vi "Write Sender.vi"(8 "error in (no error)":errorcluster, 10 "Sender":string, 11 "iMessage in":refnum<class "iMessage.lvclass">) -> (0 "error out":errorcluster, 3 "iMessage out":refnum<class "iMessage.lvclass">)   [LabVIEW 2017, in "Message Interface.lvlib" / "iMessage.lvclass"]
uses:
  iMessage.lvclass
  iMessage.lvclass/iMessage.ctl
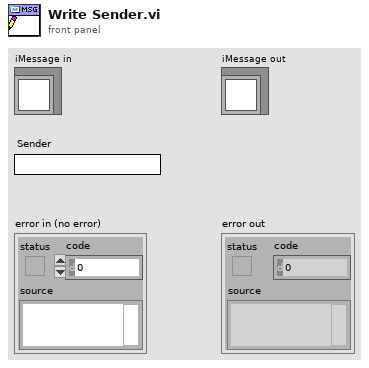
[diagram p1: front panel]
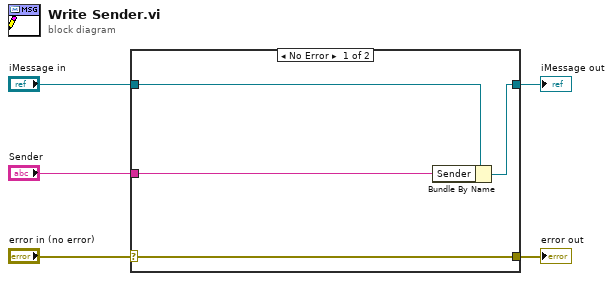
[diagram p0: block diagram]
diagram:
  n1 = case shown="No Error" "error in (no error)" {
    selector: "error in (no error)" -> [w9 w10]
    tunnel: [w9 w10] -> w4
    tunnel: [w7 w11] -> w2
    tunnel: "iMessage in" -> [w8 w11]
    tunnel: "Sender" -> [w6 _]
    frame No Error {
      n2 = Bundle By Name(cluster=w8, "Sender"=w6) -> (w7:refnum<class "iMessage.lvclass">)
    }
    frame Error {
    }
  }
  "error out" <- w4
  "iMessage out" <- w2
